vi "DPD Apply.vi"(0 "RFmx Handle In":refnum<k21>, 1 "Selector String":string, 5 "Waveform to Predistort":T1={"Waveform"={"x0"=0.0, "dx"=0.0, "y"=[]}, "Idle Duration Present"=0, "PAPR (dB)"=0.0, "Waveform Name"="Wfm"} {"PAPR (dB)" format="%.2f"; "Idle Duration Present" items=["False", "True"]; "Waveform"."y" format="%.2f"; "Waveform"."dx" format="%^.2e"; "Waveform"."x0" format="%^.2e"}, 11 "error in (no error)":errorcluster) -> (4 "RFmx Handle Out":refnum<k21>, 6 "Predistorted Waveform":T1={"Waveform"={"x0"=0.0, "dx"=0.0, "y"=[]}, "Idle Duration Present"=0, "PAPR (dB)"=0.0, "Waveform Name"="Wfm"} {"PAPR (dB)" format="%.2f"; "Idle Duration Present" items=["False", "True"]; "Waveform"."y" format="%.2f"; "Waveform"."dx" format="%^.2e"; "Waveform"."x0" format="%^.2e"}, 15 "error out":errorcluster)   [LabVIEW 2018, in "RFmxSpecAn.lvlib"]
uses:
  RFmxSpecAn.lvlib
  SG/Typedefs/Waveform.ctl
  SG/SG.lvlib
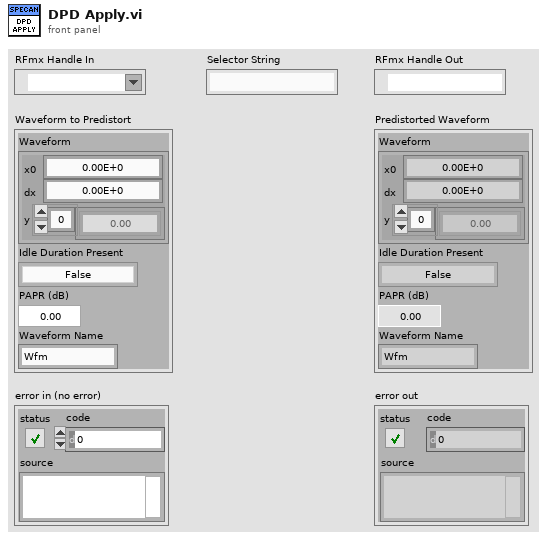
[diagram p1: front panel]
types:
  T1 = typedef "SG.lvlib/Waveform.ctl" = cluster{"Waveform":cluster{"x0":dbl, "dx":dbl, "y":csg[]}, "Idle Duration Present":i32, "PAPR (dB)":dbl, "Waveform Name":string}
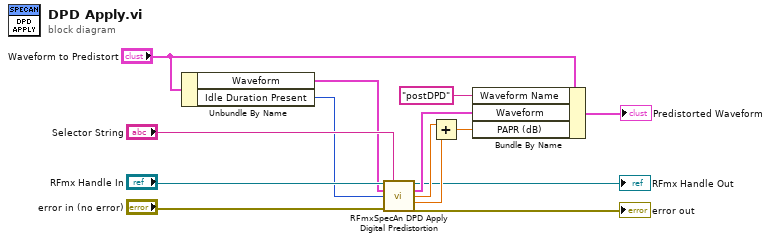
[diagram p0: block diagram]
diagram:
  n1 = Unbundle By Name("Waveform to Predistort") -> ("Waveform"=w6:cluster{"x0":dbl, "dx":dbl, "y":csg[]}, "Idle Duration Present"=w5:i32)
  n2 = call <vilib>:"RFmxSpecAn DPD Apply Digital Predistortion.vi"("Instrument Handle In"="RFmx Handle In", "Selector String"="Selector String", "Waveform In"=w6, "Idle Duration Present"=w5, "error in (no error)"="error in (no error)") -> ("Instrument Handle Out"=→"RFmx Handle Out":refnum<k21>, "Waveform Out"=w14:cluster{"x0":dbl, "dx":dbl, "y":csg[]}, "PAPR (dB)"=w13:dbl, "Power Offset (dB)"=w12:dbl, "error out"=→"error out":errorcluster)  [unwired: 6 in]
  n3 = Add(x=w13, y=w12) -> (x+y=w11:dbl)
  n4 = Bundle By Name(cluster="Waveform to Predistort", "Waveform Name"="postDPD", "Waveform"=w14, "PAPR (dB)"=w11) -> (→"Predistorted Waveform":T1)
